vi "Fast spectrum measurment.vi"() -> ()   [LabVIEW 2020]
panel:
  in  "Stop 2":bool
  out "XY Graph":T1(graph)
  out "Spectrum Values":dbl[](array[numeric])
  out "WL Values":dbl[](array[numeric])
  out "ContinuousStrobe Out":u32
  in  "conous strobe delay":i32
  in  "Enter the \nInetegration Time":i32
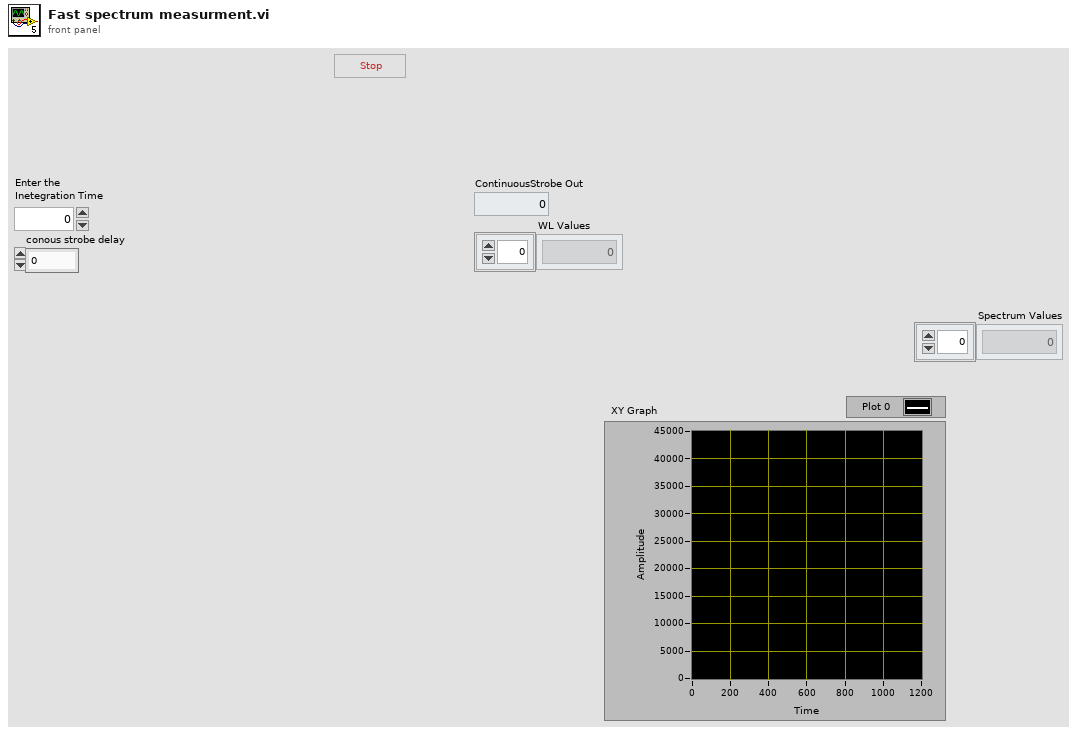
[diagram p1: front panel]
types:
  T1 = cluster{"WL Values":dbl[], "Spectrum Values":dbl[]}
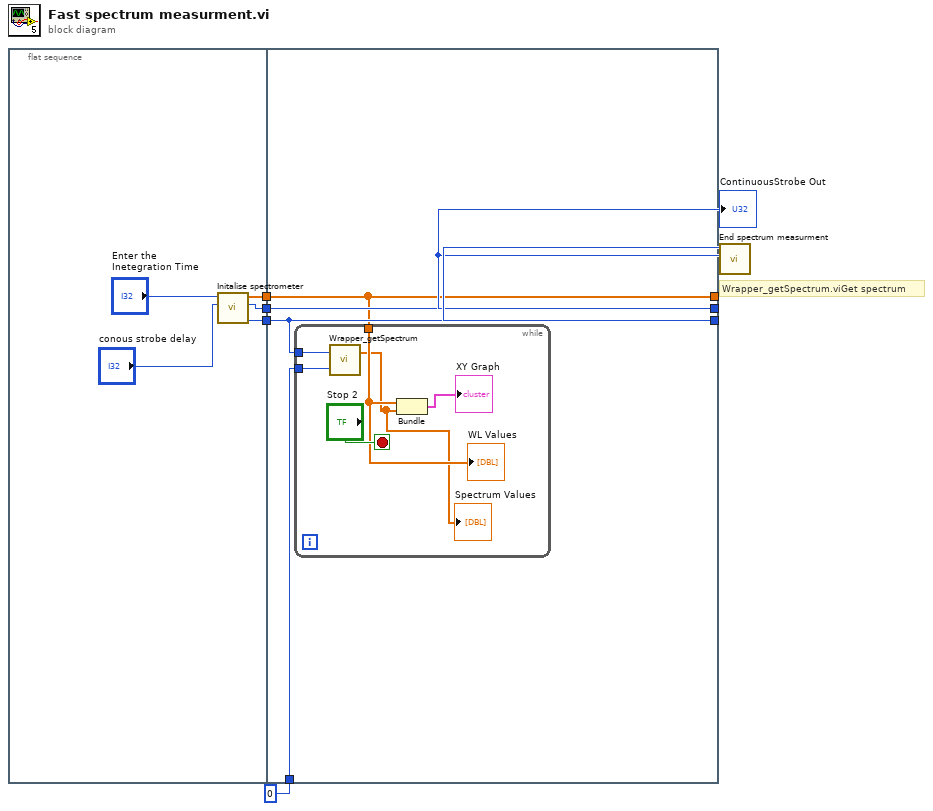
[diagram p0: block diagram]
diagram:
  # "Wrapper_getSpectrum.viGet spectrum"
  n1 = flat-sequence {
    tunnel: [w9] -> w6
    tunnel: [w8] -> w5
    tunnel: [w7] -> w4
    tunnel: [w14] -> w2
    tunnel: [w15] -> w3
    tunnel: [w12] -> _
    tunnel: w6 -> [w12]
    tunnel: w5 -> [w15]
    tunnel: w4 -> [w14]
    tunnel: 0 ("Index") -> [w13]
    frame #0 {
      n2 = call "Initalise spectrometer.vi"("conous strobe delay"="conous strobe delay", "Enter the \nInetegration Time"="Enter the \nInetegration Time") -> ("Wrapper Out"=w8:u32, "ContinuousStrobe Out"=w7:u32, "WL Values"=w9:dbl[])  [unwired: 7 in]
    }
    frame #1 {
      n3 = while {
        tunnel: w15 -> [w21]
        tunnel: w13 -> [w20]
        tunnel: w12 -> [w17]
        stop <- "Stop 2" stop-if-true
        n4 = call "Wrapper_getSpectrum.vi"("Index"=w20, "Wrapper"=w21) -> ("Spectrum Values"=w16:dbl[])  [unwired: 1 out]
        "Spectrum Values" <- w16
        n5 = Bundle("WL Values"=w17, "Spectrum Values"=w16) -> (→"XY Graph":T1)  [unwired: 1 in]
        "WL Values" <- w17
      }
    }
  }
  n6 = call "End spectrum measurment.vi"("ContinuousStrobe Out"=w2, "Wrapper Out"=w3) -> ()  [unwired: 10 in]
  "ContinuousStrobe Out" <- w2
